vi "Mouse Wheel Scroll Event.vi"(8 "错误输入（无错误）":errorcluster, 11 "dwData":i32) -> (0 "错误输出":errorcluster)   [LabVIEW 2012, in "API.lvlib"]
uses:
  API.lvlib
  Mouse_Event.ctl
  user32.dll
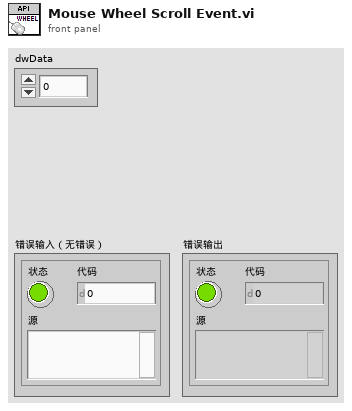
[diagram p1: front panel]
types:
  T1 = typedef "API.lvlib/Mouse_Event.ctl" = u32
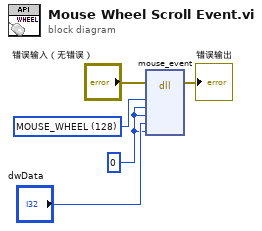
[diagram p0: block diagram]
diagram:
  w1 = u32 0 ("dwExtraInfo")
  w5 = T1 128 items=["MOVE"=1, "LEFT_DOWN"=2, "lEFT_UP"=4, "RIGHT_DOWN"=8, "RIGHT_UP"=16, "MIDDLE_DOWN"=32, "MIDDLE_UP"=64, "MOUSE_WHEEL"=128, "ABSOLUTE"=32768] ("文本下拉列表")
  n1 = dll-call lib="user32.dll" fn="mouse_event"(error in="错误输入（无错误）", "dwFlags"=w5, "dx"=w1, "dy"=w1, "dwData"="dwData", "dwExtraInfo"=w1) -> (error out=→"错误输出":errorcluster)  [unwired: 8 in, 1 out]
